vi "Initial CardClass.vi"(7 "Enum":enum16{"Initial", "Write", "Read", "Exit"}(ring)=enum."Exit", 8 "error in":errorcluster, 10 "Card Number":i32, 11 "ClassIn":refnum<class "AxisCard.lvclass">) -> (0 "error Out":errorcluster, 3 "DataOut":refnum<class "AxisCard.lvclass">)   [LabVIEW 2019, in "AxisCard.lvclass"]
uses:
  AxisCard.lvclass
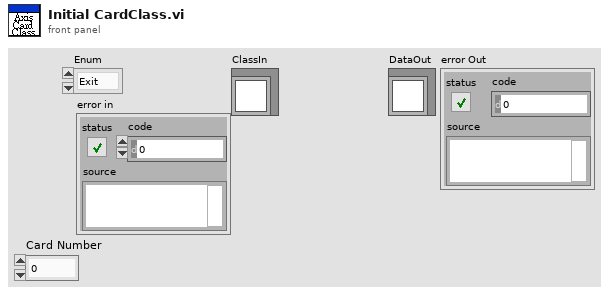
[diagram p1: front panel]
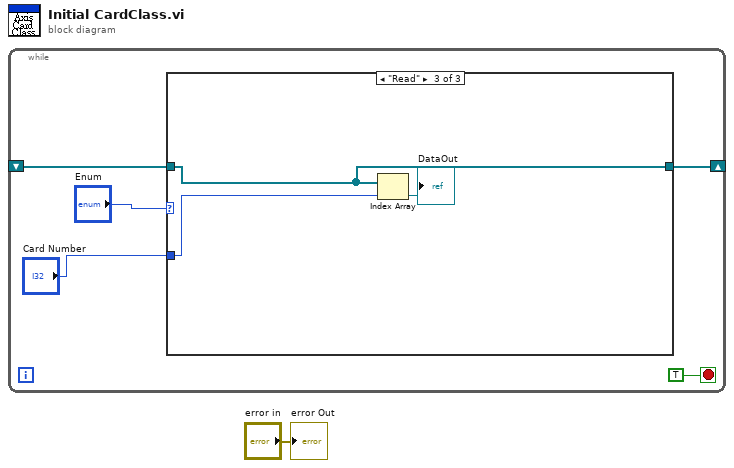
[diagram p0: block diagram]
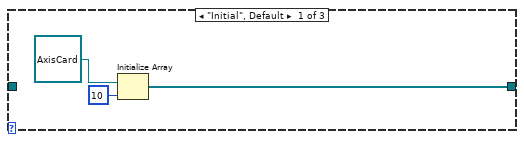
[diagram p2: hidden frame]
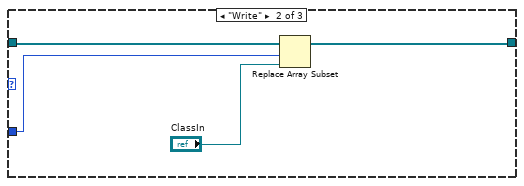
[diagram p3: hidden frame]
diagram:
  n1 = while {
    shift-right: [w5] -> _
    shift-left: _ -> [w4]
    stop <- TRUE stop-if-true
    n2 = case shown="\"Read\"" "Enum" {
      tunnel: [w7 w12 w15] -> w5
      tunnel: w4 -> [_ w13 w15]
      tunnel: "Card Number" -> [_ w10 w16]
      frame "Initial", Default {
        n3 = Initialize Array(refnum<class "AxisCard.lvclass"> refnum ("AxisCard out"), 10 ("dimension size")) -> (w7:refnum<class "AxisCard.lvclass">[])
      }
      frame "Write" {
        n4 = Replace Array Subset(array=w13, new element="ClassIn", index=w10) -> (w12:refnum<class "AxisCard.lvclass">[])
      }
      frame "Read" {
        n5 = Index Array(array=w15, index=w16) -> (element=→"DataOut":refnum<class "AxisCard.lvclass">)
      }
    }
  }
  "error Out" <- "error in"
